vi "Process.vi"(8 "error in (no error)":errorcluster, 9 "Panel":refnum<class "Panel Controller Interface.lvclass">, 10 "Console Reply.lvclass":refnum<class "Console Reply.lvclass">, 11 "Delete Control In Panel_Msg":refnum<class "Delete Control_Behavior.lvclass">) -> (0 "error out":errorcluster, 3 "Delete Control In Panel_Msg":refnum<class "Delete Control_Behavior.lvclass">)   [LabVIEW 2015, in "Delete Control_Behavior.lvclass"]
uses:
  Delete Control_Behavior.lvclass
  _Depences/Panel API/Console Reply/Console Reply/Console Reply.lvclass
  _Depences/Panel API/Panel Control_Interface/Panel_interface/Panel Controller Interface.lvclass
  _Depences/Panel API/Console Reply/Console Reply/Console Reply.lvclass/Console Reply.ctl
  Delete Control_Behavior.lvclass/Delete Control_Behavior.ctl
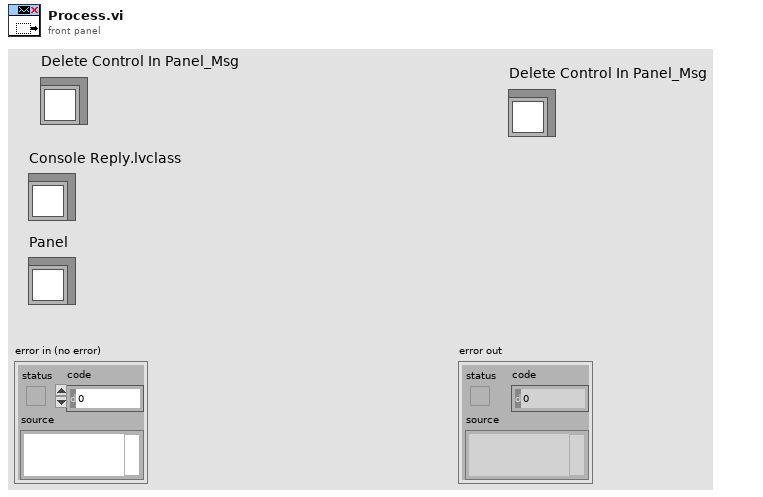
[diagram p1: front panel]
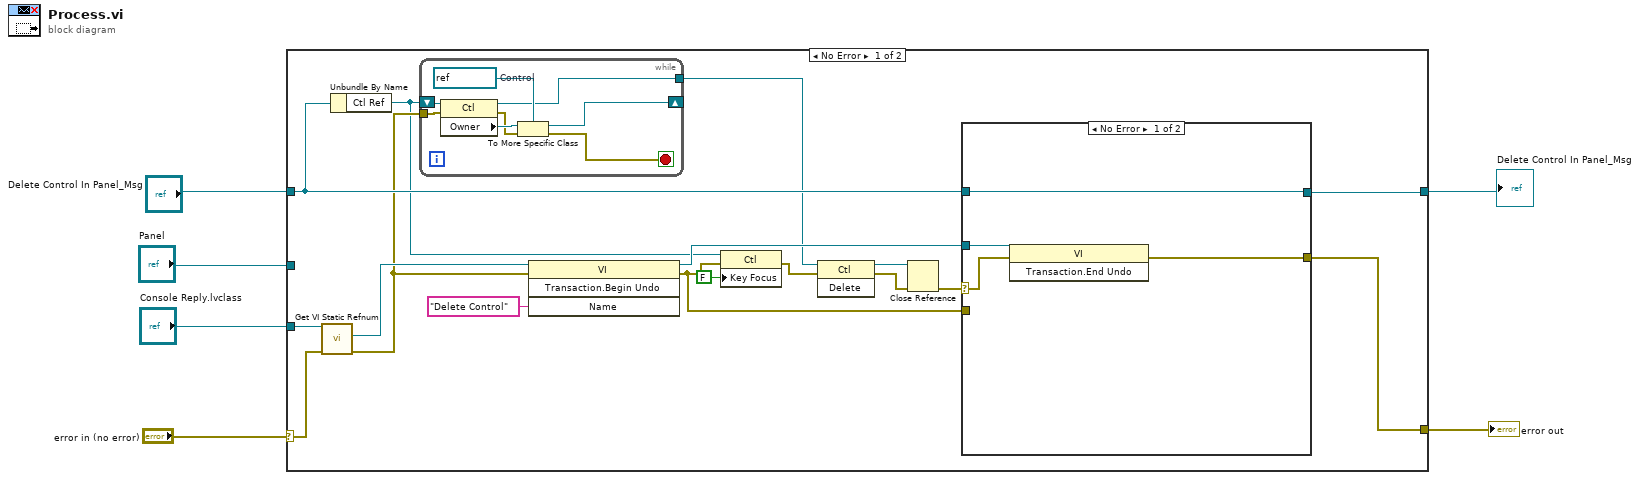
[diagram p0: block diagram]
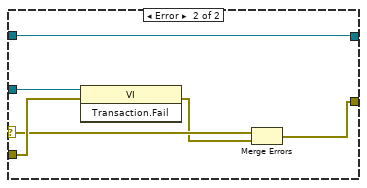
[diagram p2: hidden frame]
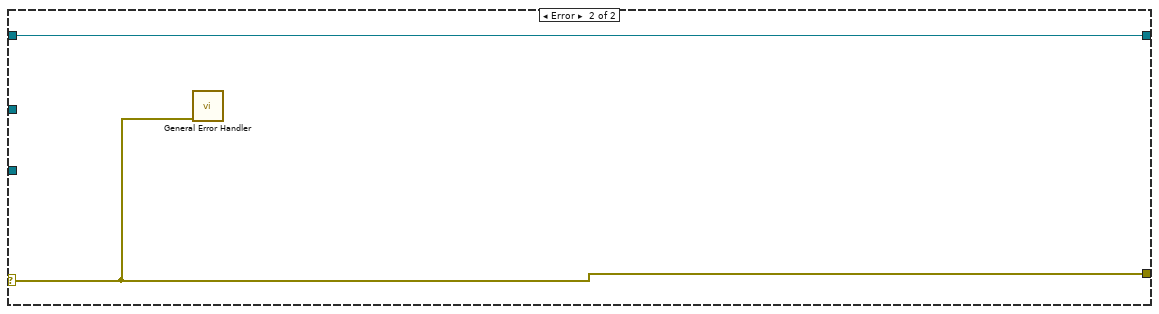
[diagram p3: hidden frame]
diagram:
  n1 = case shown="No Error" "error in (no error)" {
    selector: "error in (no error)" -> [w14 w42]
    tunnel: [w17 w42] -> w5
    tunnel: [w18 w43] -> w3
    tunnel: "Delete Control In Panel_Msg" -> [w16 w43]
    tunnel: "Console Reply.lvclass" -> [w15 _]
    tunnel: "Panel" -> [_ _]
    frame No Error {
      n2 = call "Get VI Static Refnum.vi"("error in (no error)"=w14, "Console Reply in"=w15) -> ("error out"=w12:errorcluster, "VI Static Refnum"=w13:refnum<vi>)  [unwired: 7 in, 1 out]
      n3 = Unbundle By Name(w16) -> ("Ctl Ref"=w11:refnum<vi>)
      n4 = while {
        tunnel: w12 -> [w30]
        shift-right: [w25] -> _
        shift-left: w11 -> [w31]
        tunnel: [w24] -> w8
        stop <- w26 stop-if-true
        w28 = refnum<vi> refnum  # Control
        n5 = property class="Ctl"(reference=w31, error in=w30) -> (reference out=w24:refnum<vi>, error out=w27:errorcluster, "Owner"=w29:refnum<vi>)
        n6 = To More Specific Class(target class=w28, reference=w29, error in=w27) -> (specific class reference=w25:refnum<vi>, error out=w26:errorcluster)
      }
      n7 = invoke class="VI" method="Transaction.Begin Undo"(reference=w13, error in=w12, "Name"="Delete Control") -> (reference out=w23:refnum<vi>, error out=w7:errorcluster)  [unwired: 1 in, 2 out]
      n8 = property class="Ctl"(reference=w11, error in=w7, "Key Focus"=FALSE) -> (error out=w9:errorcluster)  [unwired: 1 out]
      n9 = invoke class="Ctl" method="Delete"(reference=w8, error in=w9) -> (reference out=w20:refnum<vi>, error out=w21:errorcluster)  [unwired: 1 in, 1 out]
      n10 = Close Reference(reference=w20, error in (no error)=w21) -> (error out=w22:errorcluster)
      n11 = case shown="No Error" w22 {
        selector: w22 -> [w34 w39]
        tunnel: [w33 w37] -> w17
        tunnel: w23 -> [w35 w41]
        tunnel: w7 -> [_ w40]
        tunnel: [w32 w36] -> w18
        tunnel: w16 -> [w32 w36]
        frame No Error {
          n12 = invoke class="VI" method="Transaction.End Undo"(reference=w35, error in=w34) -> (error out=w33:errorcluster)  [unwired: 1 in, 2 out]
        }
        frame Error {
          n13 = invoke class="VI" method="Transaction.Fail"(reference=w41, error in=w40) -> (error out=w38:errorcluster)  [unwired: 1 in, 2 out]
          n14 = Merge Errors(w39, w38) -> (w37:errorcluster)
        }
      }
    }
    frame Error {
      n15 = call <vilib>:"General Error Handler.vi"("error in (no error)"=w42) -> ()  [unwired: 10 in, 5 out]
    }
  }
  "error out" <- w5
  "Delete Control In Panel_Msg" <- w3
